vi "Read Parameter.vi"(8 "error in (no error)":errorcluster, 11 "Stream in":refnum<class "Stream.lvclass">) -> (0 "error out":errorcluster, 2 "parameter":string, 3 "Stream out":refnum<class "Stream.lvclass">)   [LabVIEW 2018, in "Stream.lvclass"]
uses:
  Stream.lvclass
  Stream.lvclass/Stream.ctl
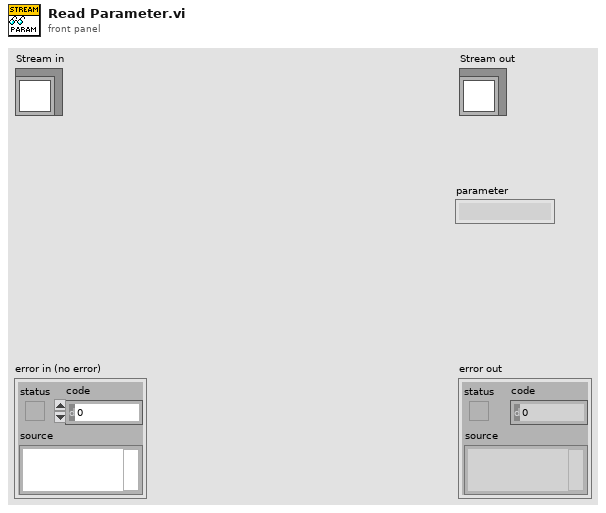
[diagram p1: front panel]
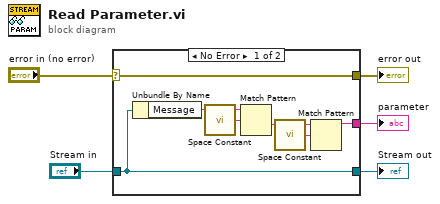
[diagram p0: block diagram]
diagram:
  n1 = case shown="No Error" "error in (no error)" {
    selector: "error in (no error)" -> [w12 w14]
    tunnel: [w12 w14] -> w4
    tunnel: [w11 w13] -> w2
    tunnel: "Stream in" -> [w11 w13]
    tunnel: [w6 _] -> w1
    frame No Error {
      n2 = Unbundle By Name(w11) -> ("Message"=w10:string)
      n3 = call <vilib>:"Space Constant.vi"() -> ("String"=w9:string)
      n4 = Match Pattern(string=w10, regular expression=w9) -> (after substring=w7:string)  [unwired: 1 in, 3 out]
      n5 = call <vilib>:"Space Constant.vi"() -> ("String"=w8:string)
      n6 = Match Pattern(string=w7, regular expression=w8) -> (before substring=w6:string)  [unwired: 1 in, 3 out]
    }
    frame Error {
    }
  }
  "error out" <- w4
  "Stream out" <- w2
  "parameter" <- w1
